vi "torrehanoi.vi"() -> ()   [LabVIEW 2020]
uses:
  <vilib>/Utility/miscctls.llb/LVPoint32TypeDef.ctl
  <vilib>/Utility/miscctls.llb/LVBoundsTypeDef.ctl
panel:
  in  "Number of Plates":i32=3
  in  "Numeros de discos":u16(ring) items=["3 Discos", "4 Discos", "5 Discos", ""]
  in  "Solucion":string
  in  "Resultado":string
  out "Torre de destino":string="Right"
  out "Torre del medio":string="Middle"
  out "Torre de origen":string="Left"
  out "Coords":T1
  out "disco5":bool
  out "disco4":bool
  out "disco3":bool
  out "disco2":bool
  out "disco1":bool
  out "final":bool
  out "medio":bool
  out "inicio":bool
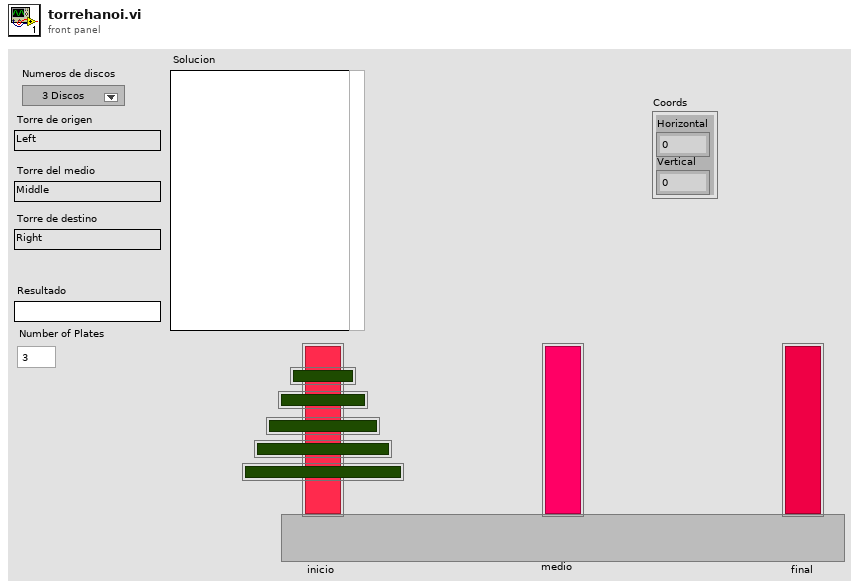
[diagram p1: front panel]
types:
  T1 = typedef "LVPoint32TypeDef.ctl" = cluster{"Horizontal":i32, "Vertical":i32}
  T2 = typedef "LVBoundsTypeDef.ctl" = cluster{"Width":u32, "Height":u32}
  T3 = typedef "LVPositionTypeDef.ctl" = cluster{"Left":i32, "Top":i32}
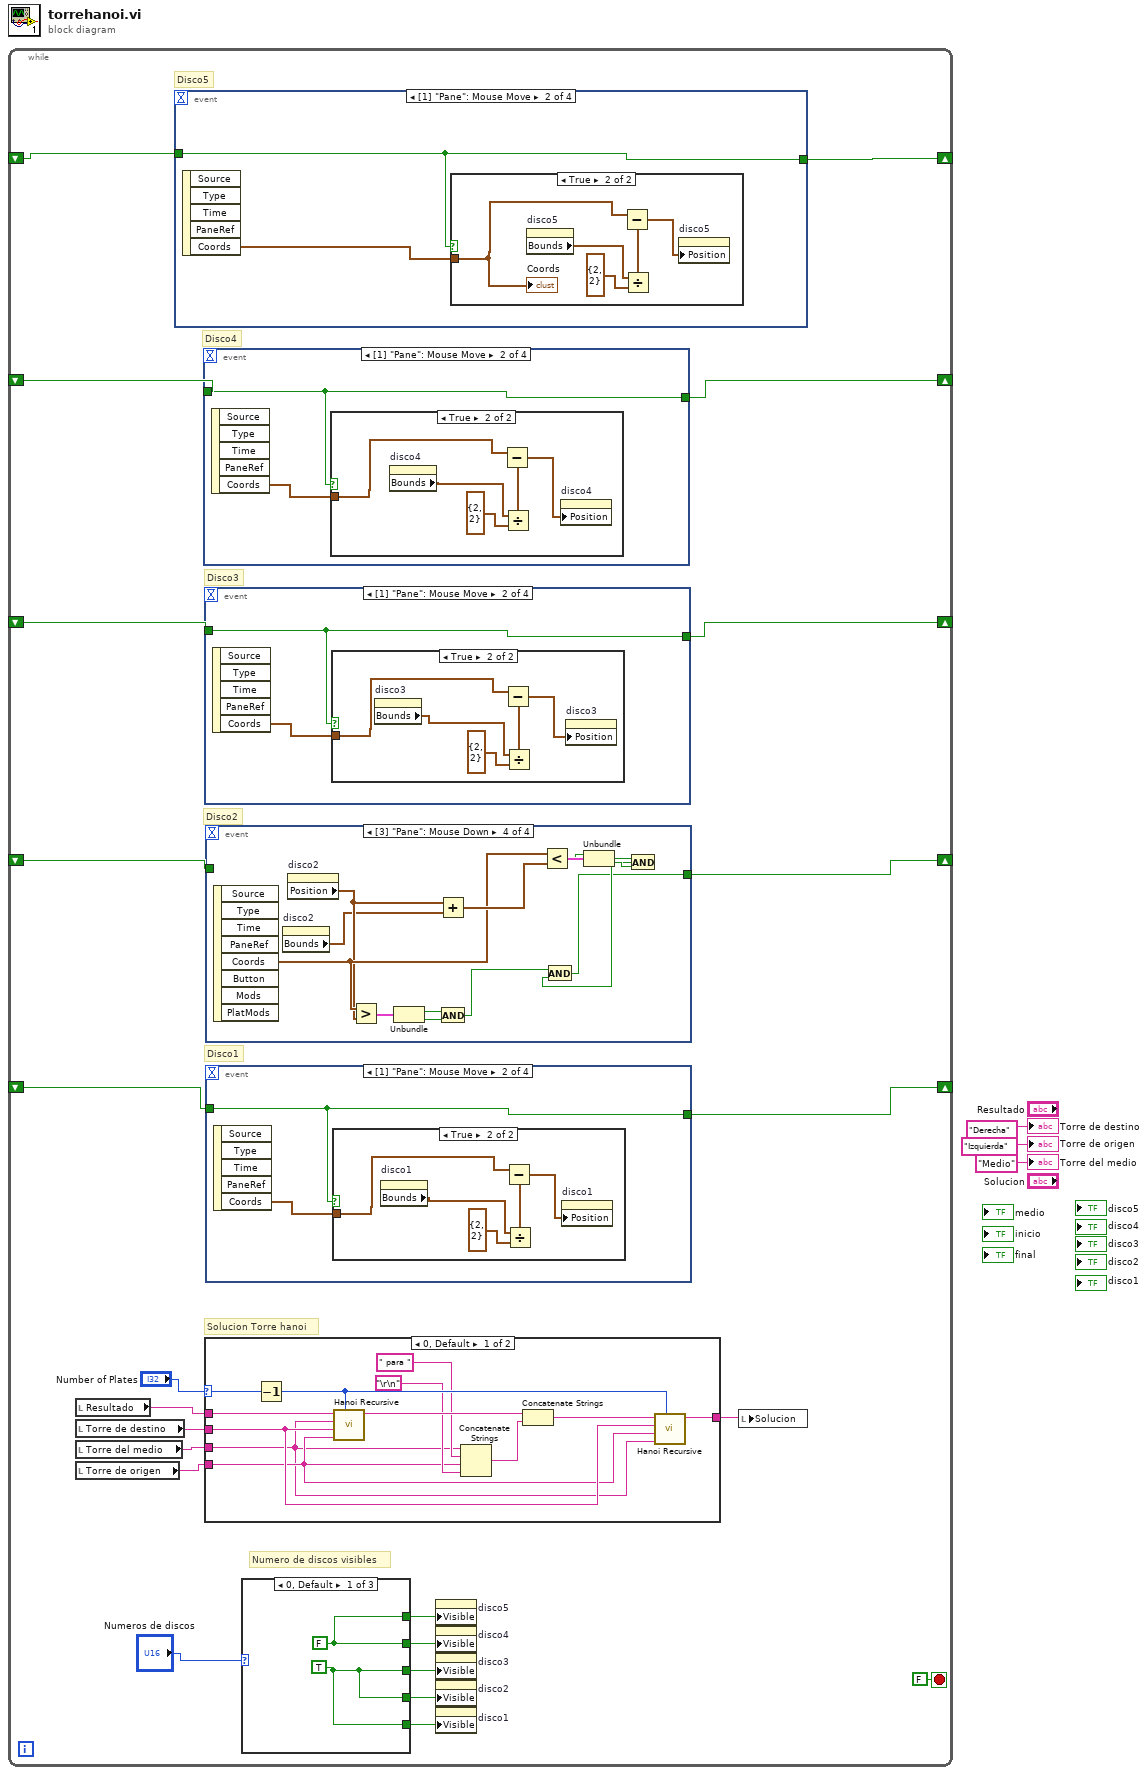
[diagram p0: block diagram]
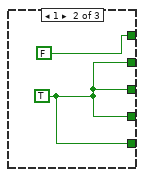
[diagram p2: hidden frame]
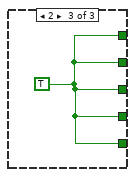
[diagram p3: hidden frame]
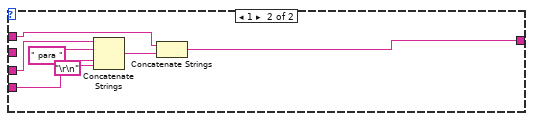
[diagram p4: hidden frame]
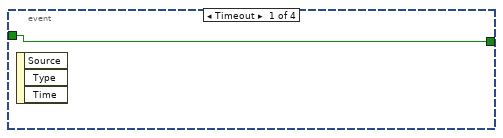
[diagram p5: hidden frame]
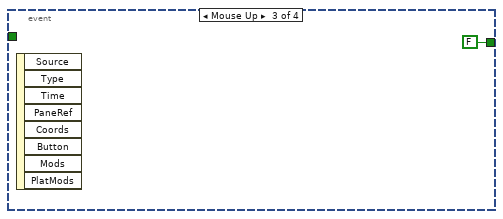
[diagram p7: hidden frame]
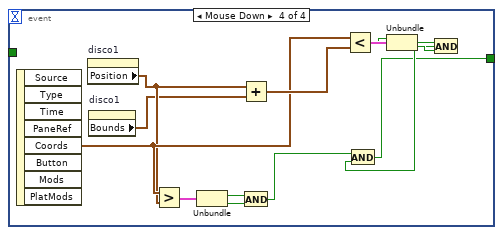
[diagram p8: hidden frame]
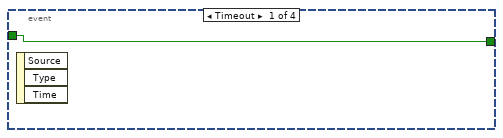
[diagram p9: hidden frame]
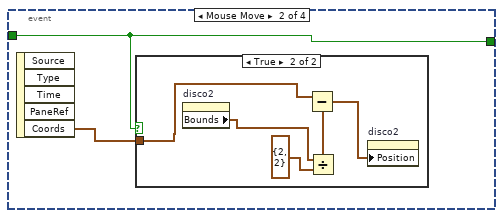
[diagram p10: hidden frame]
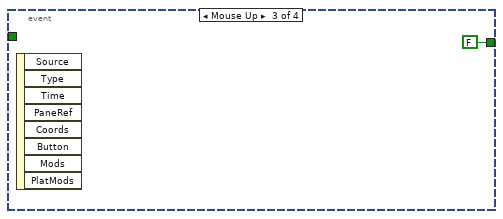
[diagram p12: hidden frame]
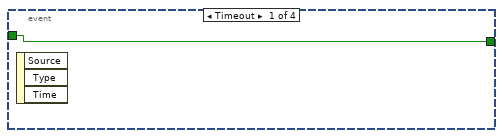
[diagram p13: hidden frame]
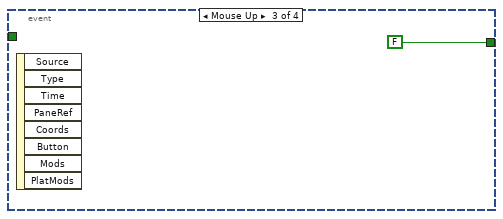
[diagram p15: hidden frame]
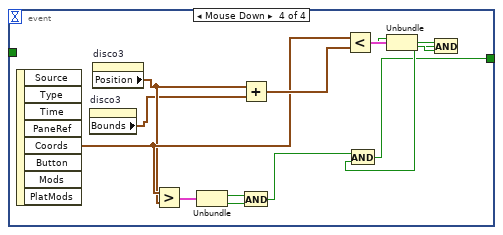
[diagram p16: hidden frame]
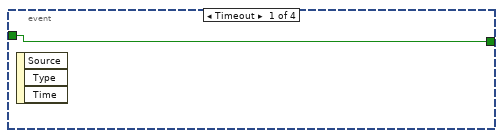
[diagram p17: hidden frame]
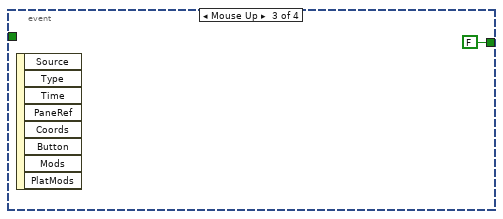
[diagram p19: hidden frame]
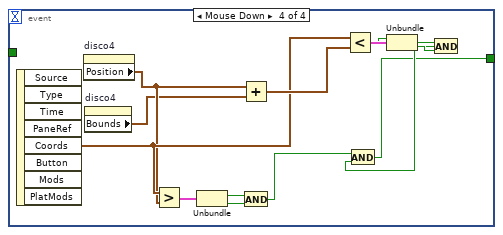
[diagram p20: hidden frame]
diagram:
  n1 = while {
    shift-right: [w24] -> _
    shift-left: _ -> [w25]
    shift-right: [w22] -> _
    shift-left: _ -> [w23]
    shift-right: [w20] -> _
    shift-left: _ -> [w21]
    shift-right: [w18] -> _
    shift-left: _ -> [w19]
    shift-right: [w16] -> _
    shift-left: _ -> [w17]
    stop <- FALSE stop-if-true
    # "Numero de discos visibles"
    # "Solucion Torre hanoi"
    # "Disco5"
    # "Disco4"
    # "Disco3"
    # "Disco2"
    # "Disco1"
    n2 = local read "Resultado"() -> (w11:string)
    n3 = local read "Torre de destino"() -> (w14:string)
    n4 = local read "Torre del medio"() -> (w13:string)
    n5 = local read "Torre de origen"() -> (w12:string)
    n6 = event shown="[1] \"Pane\": Mouse Move" {
      selector: _ -> [_ _ _ _]
      dyn-events: _ -> [_ _ _ _]
      timeout: _ -> [_ _ _ _]
      tunnel: w25 -> [w139 w140 _ _]
      tunnel: [w139 w140 FALSE w148] -> w24
      event Timeout {
        n7 = event-data() -> ()  [unwired: 1 in, 3 out]
      }
      event Mouse Move {
        n8 = event-data() -> ("Coords"=w141:T1)  [unwired: 1 in, 4 out]
        n9 = case shown="True" w140 {
          tunnel: w141 -> [_ w144]
          frame False {
          }
          frame True {
            n10 = property on="disco5" class="Bool (strict)"() -> ("Bounds"=w146:T2)  [unwired: 2 in, 2 out]
            n11 = Divide(x=w146, y=T2 {"Width"=2, "Height"=2}) -> (x/y=w143:cluster{"Width":dbl, "Height":dbl})
            n12 = Subtract(x=w144, y=w143) -> (x-y=w142:cluster{dbl, dbl})
            n13 = property on="disco5" class="Bool (strict)"("Position"=w142) -> ()  [unwired: 2 in, 2 out]
            "Coords" <- w144
          }
        }
      }
      event Mouse Up {
        n14 = event-data() -> ()  [unwired: 1 in, 8 out]
      }
      event Mouse Down {
        n15 = event-data() -> ("Coords"=w157:T1)  [unwired: 1 in, 7 out]
        n16 = property on="disco5" class="Bool (strict)"() -> ("Position"=w159:T3)  [unwired: 2 in, 2 out]
        n17 = property on="disco5" class="Bool (strict)"() -> ("Bounds"=w160:T2)  [unwired: 2 in, 2 out]
        n18 = Greater?(x=w157, y=w159) -> (0:w156:cluster{bool, bool})
        n19 = Unbundle(w156) -> (w152:bool, w151:bool)
        n20 = Add(x=w159, y=w160) -> (x+y=w158:T2)
        n21 = And(x=w152, y=w151) -> (x .and. y?=w149:bool)
        n22 = Less?(x=w157, y=w158) -> (x < y?=w155:cluster{bool, bool})
        n23 = Unbundle(w155) -> (w154:bool, w153:bool)
        n24 = And(x=w154, y=w153) -> (x .and. y?=w150:bool)
        n25 = And(x=w149, y=w150) -> (x .and. y?=w148:bool)
      }
    }
    n26 = event shown="[1] \"Pane\": Mouse Move" {
      selector: _ -> [_ _ _ _]
      dyn-events: _ -> [_ _ _ _]
      timeout: _ -> [_ _ _ _]
      tunnel: w23 -> [w117 w118 _ _]
      tunnel: [w117 w118 FALSE w128] -> w22
      event Timeout {
        n27 = event-data() -> ()  [unwired: 1 in, 3 out]
      }
      event Mouse Move {
        n28 = event-data() -> ("Coords"=w119:T1)  [unwired: 1 in, 4 out]
        n29 = case shown="True" w118 {
          tunnel: w119 -> [_ w120]
          frame False {
          }
          frame True {
            n30 = property on="disco4" class="Bool (strict)"() -> ("Bounds"=w122:T2)  [unwired: 2 in, 2 out]
            n31 = Divide(x=w122, y=T2 {"Width"=2, "Height"=2}) -> (x/y=w123:cluster{"Width":dbl, "Height":dbl})
            n32 = Subtract(x=w120, y=w123) -> (x-y=w121:cluster{dbl, dbl})
            n33 = property on="disco4" class="Bool (strict)"("Position"=w121) -> ()  [unwired: 2 in, 2 out]
          }
        }
      }
      event Mouse Up {
        n34 = event-data() -> ()  [unwired: 1 in, 8 out]
      }
      event Mouse Down {
        n35 = event-data() -> ("Coords"=w137:T1)  [unwired: 1 in, 7 out]
        n36 = property on="disco4" class="Bool (strict)"() -> ("Position"=w127:T3)  [unwired: 2 in, 2 out]
        n37 = property on="disco4" class="Bool (strict)"() -> ("Bounds"=w126:T2)  [unwired: 2 in, 2 out]
        n38 = Greater?(x=w137, y=w127) -> (0:w136:cluster{bool, bool})
        n39 = Unbundle(w136) -> (w132:bool, w131:bool)
        n40 = Add(x=w127, y=w126) -> (x+y=w138:T2)
        n41 = And(x=w132, y=w131) -> (x .and. y?=w129:bool)
        n42 = Less?(x=w137, y=w138) -> (x < y?=w135:cluster{bool, bool})
        n43 = Unbundle(w135) -> (w134:bool, w133:bool)
        n44 = And(x=w134, y=w133) -> (x .and. y?=w130:bool)
        n45 = And(x=w129, y=w130) -> (x .and. y?=w128:bool)
      }
    }
    n46 = event shown="[1] \"Pane\": Mouse Move" {
      selector: _ -> [_ _ _ _]
      dyn-events: _ -> [_ _ _ _]
      timeout: _ -> [_ _ _ _]
      tunnel: w21 -> [w95 w96 _ _]
      tunnel: [w95 w96 FALSE ("Accepted?") w106] -> w20
      event Timeout {
        n47 = event-data() -> ()  [unwired: 1 in, 3 out]
      }
      event Mouse Move {
        n48 = event-data() -> ("Coords"=w97:T1)  [unwired: 1 in, 4 out]
        n49 = case shown="True" w96 {
          tunnel: w97 -> [_ w101]
          frame False {
          }
          frame True {
            n50 = property on="disco3" class="Bool (strict)"() -> ("Bounds"=w99:T2)  [unwired: 2 in, 2 out]
            n51 = Divide(x=w99, y=T2 {"Width"=2, "Height"=2}) -> (x/y=w100:cluster{"Width":dbl, "Height":dbl})
            n52 = Subtract(x=w101, y=w100) -> (x-y=w98:cluster{dbl, dbl})
            n53 = property on="disco3" class="Bool (strict)"("Position"=w98) -> ()  [unwired: 2 in, 2 out]
          }
        }
      }
      event Mouse Up {
        n54 = event-data() -> ()  [unwired: 1 in, 8 out]
      }
      event Mouse Down {
        n55 = event-data() -> ("Coords"=w115:T1)  [unwired: 1 in, 7 out]
        n56 = property on="disco3" class="Bool (strict)"() -> ("Bounds"=w104:T2)  [unwired: 2 in, 2 out]
        n57 = property on="disco3" class="Bool (strict)"() -> ("Position"=w105:T3)  [unwired: 2 in, 2 out]
        n58 = Greater?(x=w115, y=w105) -> (0:w114:cluster{bool, bool})
        n59 = Unbundle(w114) -> (w110:bool, w109:bool)
        n60 = Add(x=w105, y=w104) -> (x+y=w116:T2)
        n61 = And(x=w110, y=w109) -> (x .and. y?=w107:bool)
        n62 = Less?(x=w115, y=w116) -> (x < y?=w113:cluster{bool, bool})
        n63 = Unbundle(w113) -> (w112:bool, w111:bool)
        n64 = And(x=w112, y=w111) -> (x .and. y?=w108:bool)
        n65 = And(x=w107, y=w108) -> (x .and. y?=w106:bool)
      }
    }
    n66 = case shown="0, Default" "Number of Plates" {
      selector: "Number of Plates" -> [w43 _]
      tunnel: w13 -> [w32 w50]
      tunnel: w14 -> [w34 _]
      tunnel: w12 -> [w33 w44]
      tunnel: w11 -> [w40 w47]
      tunnel: [w38 w45] -> w15
      frame 0, Default {
        n67 = Decrement(x=w43) -> (x-1=w42:i32)
        n68 = call "Hanoi Recursive.vi"("Number of Plates"=w42, "Torre de destino"=w33, "Torre del medio"=w34, "Torre de origen"=w32, "Resultado"=w40) -> ("Solution"=w39:string)  [unwired: 6 in]
        n69 = Concatenate Strings(w32, " para ", w33, "\r\n") -> (w41:string)
        n70 = Concatenate Strings(w39, w41) -> (w35:string)
        n71 = call "Hanoi Recursive.vi"("Number of Plates"=w42, "Torre de destino"=w32, "Torre del medio"=w33, "Torre de origen"=w34, "Resultado"=w35) -> ("Solution"=w38:string)  [unwired: 6 in]
      }
      frame 1 {
        n72 = Concatenate Strings(w50, " para ", w44, "\r\n") -> (w46:string)
        n73 = Concatenate Strings(w47, w46) -> (w45:string)
      }
    }
    n74 = event shown="[3] \"Pane\": Mouse Down" {
      selector: _ -> [_ _ _ _]
      dyn-events: _ -> [_ _ _ _]
      timeout: _ -> [_ _ _ _]
      tunnel: w19 -> [w73 w74 _ _]
      tunnel: [w73 w74 FALSE w84] -> w18
      event Timeout {
        n75 = event-data() -> ()  [unwired: 1 in, 3 out]
      }
      event Mouse Move {
        n76 = event-data() -> ("Coords"=w75:T1)  [unwired: 1 in, 4 out]
        n77 = case shown="True" w74 {
          tunnel: w75 -> [_ w79]
          frame False {
          }
          frame True {
            n78 = property on="disco2" class="Bool (strict)"() -> ("Bounds"=w77:T2)  [unwired: 2 in, 2 out]
            n79 = Divide(x=w77, y=T2 {"Width"=2, "Height"=2}) -> (x/y=w78:cluster{"Width":dbl, "Height":dbl})
            n80 = Subtract(x=w79, y=w78) -> (x-y=w76:cluster{dbl, dbl})
            n81 = property on="disco2" class="Bool (strict)"("Position"=w76) -> ()  [unwired: 2 in, 2 out]
          }
        }
      }
      event Mouse Up {
        n82 = event-data() -> ()  [unwired: 1 in, 8 out]
      }
      event Mouse Down {
        n83 = event-data() -> ("Coords"=w93:T1)  [unwired: 1 in, 7 out]
        n84 = property on="disco2" class="Bool (strict)"() -> ("Bounds"=w82:T2)  [unwired: 2 in, 2 out]
        n85 = property on="disco2" class="Bool (strict)"() -> ("Position"=w83:T3)  [unwired: 2 in, 2 out]
        n86 = Greater?(x=w93, y=w83) -> (0:w92:cluster{bool, bool})
        n87 = Unbundle(w92) -> (w88:bool, w87:bool)
        n88 = Add(x=w83, y=w82) -> (x+y=w94:T2)
        n89 = And(x=w88, y=w87) -> (x .and. y?=w85:bool)
        n90 = Less?(x=w93, y=w94) -> (x < y?=w91:cluster{bool, bool})
        n91 = Unbundle(w91) -> (w90:bool, w89:bool)
        n92 = And(x=w90, y=w89) -> (x .and. y?=w86:bool)
        n93 = And(x=w85, y=w86) -> (x .and. y?=w84:bool)
      }
    }
    n94 = event shown="[1] \"Pane\": Mouse Move" {
      selector: _ -> [_ _ _ _]
      dyn-events: _ -> [_ _ _ _]
      timeout: _ -> [_ _ _ _]
      tunnel: w17 -> [w51 w52 _ _]
      tunnel: [w51 w52 FALSE w62] -> w16
      event Timeout {
        n95 = event-data() -> ()  [unwired: 1 in, 3 out]
      }
      event Mouse Move {
        n96 = event-data() -> ("Coords"=w53:T1)  [unwired: 1 in, 4 out]
        n97 = case shown="True" w52 {
          tunnel: w53 -> [_ w57]
          frame False {
          }
          frame True {
            n98 = property on="disco1" class="Bool (strict)"() -> ("Bounds"=w55:T2)  [unwired: 2 in, 2 out]
            n99 = Divide(x=w55, y=T2 {"Width"=2, "Height"=2}) -> (x/y=w56:cluster{"Width":dbl, "Height":dbl})
            n100 = Subtract(x=w57, y=w56) -> (x-y=w54:cluster{dbl, dbl})
            n101 = property on="disco1" class="Bool (strict)"("Position"=w54) -> ()  [unwired: 2 in, 2 out]
          }
        }
      }
      event Mouse Up {
        n102 = event-data() -> ()  [unwired: 1 in, 8 out]
      }
      event Mouse Down {
        n103 = event-data() -> ("Coords"=w71:T1)  [unwired: 1 in, 7 out]
        n104 = property on="disco1" class="Bool (strict)"() -> ("Position"=w61:T3)  [unwired: 2 in, 2 out]
        n105 = property on="disco1" class="Bool (strict)"() -> ("Bounds"=w60:T2)  [unwired: 2 in, 2 out]
        n106 = Greater?(x=w71, y=w61) -> (0:w70:cluster{bool, bool})
        n107 = Unbundle(w70) -> (w66:bool, w65:bool)
        n108 = Add(x=w61, y=w60) -> (x+y=w72:T2)
        n109 = And(x=w66, y=w65) -> (x .and. y?=w63:bool)
        n110 = Less?(x=w71, y=w72) -> (x < y?=w69:cluster{bool, bool})
        n111 = Unbundle(w69) -> (w68:bool, w67:bool)
        n112 = And(x=w68, y=w67) -> (x .and. y?=w64:bool)
        n113 = And(x=w63, y=w64) -> (x .and. y?=w62:bool)
      }
    }
    n114 = case shown="0, Default" "Numeros de discos" {
      tunnel: [w28 FALSE w31] -> w10
      tunnel: [w28 w30 w31] -> w9
      tunnel: [w27 w30 w31] -> w8
      tunnel: [w27 w30 w31] -> w7
      tunnel: [w27 w30 w31] -> w6
      frame 0, Default {
        w28 = FALSE
        w27 = TRUE
      }
      frame 1 {
        w30 = TRUE
      }
      frame 2 {
        w31 = TRUE
      }
    }
    n115 = property on="disco5" class="Bool (strict)"("Visible"=w10) -> ()  [unwired: 2 in, 2 out]
    n116 = property on="disco4" class="Bool (strict)"("Visible"=w9) -> ()  [unwired: 2 in, 2 out]
    n117 = property on="disco3" class="Bool (strict)"("Visible"=w8) -> ()  [unwired: 2 in, 2 out]
    n118 = property on="disco2" class="Bool (strict)"("Visible"=w7) -> ()  [unwired: 2 in, 2 out]
    n119 = property on="disco1" class="Bool (strict)"("Visible"=w6) -> ()  [unwired: 2 in, 2 out]
    n120 = local write "Solucion"(w15) -> ()
  }
  "Torre de origen" <- "Izquierda" ("Torre de destino")
  "Torre del medio" <- "Medio" ("Torre de destino")
  "Torre de destino" <- "Derecha" ("Torre de destino")
